vi "SR Test Launcher.vi"() -> ()   [LabVIEW 2018]
doc: "This VI is the launcher for the Car Wash Simulator.\n\nThis VI performs any actions required to occur before the modules begin running or after they close \n(such as creating the user events). \nIt then launches the modules. The UI is launched dynamically when the program is run."
uses:
  User Events/controls/Actions.ctl
  Modules/Error Handler/Error Handler.lvlib
  Modules/Base Controller/Controller.lvlib
  Modules/Database/Database.lvlib
panel:
  out "progress":u32(slide) scale=0.0..1500.0
  in  "error in":errorcluster
  out "error out":errorcluster
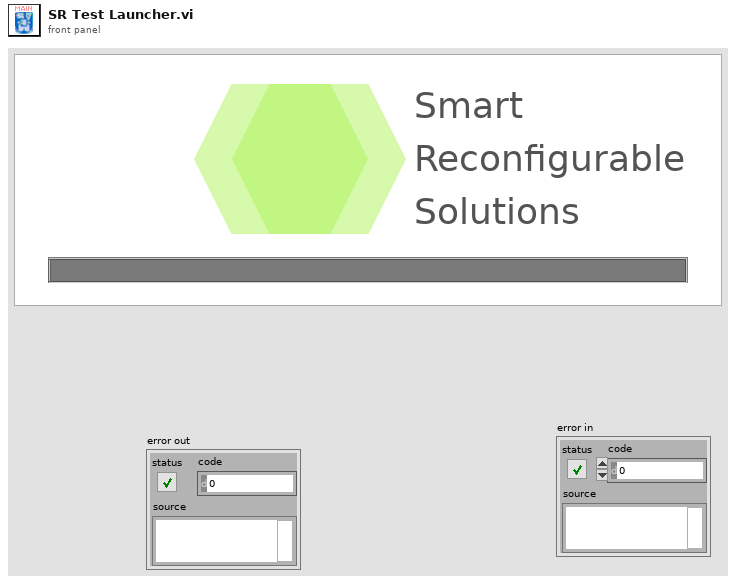
[diagram p1: front panel]
types:
  T1 = enum32{"Invalid", "Standard", "Closed", "Hidden", "Minimized", "Maximized"}
  T2 = typedef "Actions.ctl" = enum16{"Get", "Create", "Destroy"}
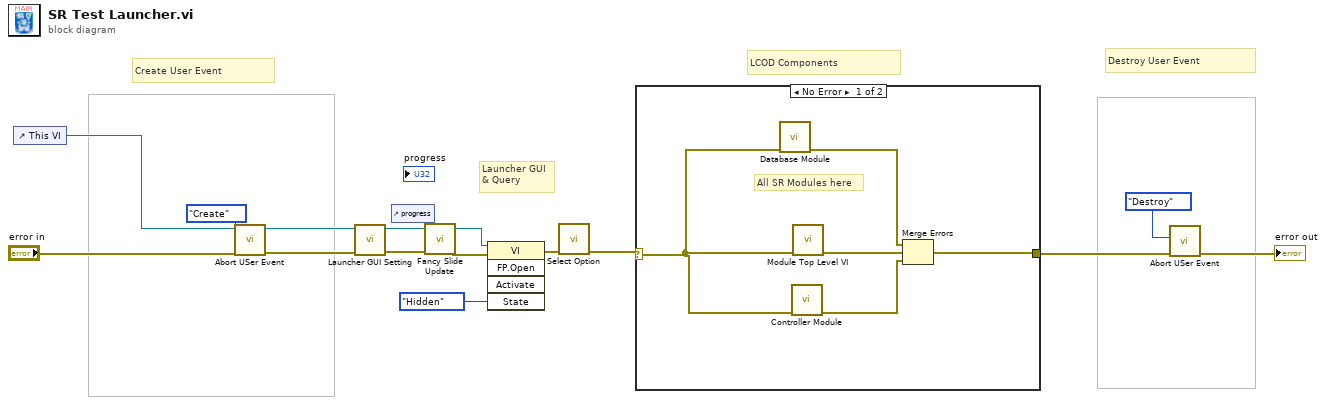
[diagram p0: block diagram]
diagram:
  # "Destroy User Event"
  # "LCOD Components"
  # "Create User Event"
  # "Launcher GUI\n& Query"
  n1 = control-ref of="This VI"() -> (w9:refnum<vi>)
  n2 = call "Abort USer Event.vi"("error in"="error in", "Enum"=Actions."Create") -> ("error out"=w10:errorcluster)  [unwired: 8 in, 1 out]
  n3 = call "Launcher GUI Setting.vi"("error in (no error)"=w10, "VI in"=w9) -> ("error out"=w6:errorcluster, "VI out"=w7:refnum<vi>)  [unwired: 8 in]
  n4 = control-ref of="progress"() -> (w4:refnum<vi>)
  n5 = call "Fancy Slide Update.vi"("error in (no error)"=w6, "Slide in"=w4) -> ("error out"=w1:errorcluster)  [unwired: 9 in]
  n6 = invoke class="VI" method="FP.Open"(reference=w7, error in=w1, "State"=T1."Hidden") -> (error out=w3:errorcluster)  [unwired: 2 in, 4 out]
  n7 = call "Select Option.vi"("error in"=w3) -> ("error out"=w2:errorcluster)  [unwired: 9 in, 1 out]
  n8 = case shown="No Error" w2 {
    selector: w2 -> [w16 w20]
    tunnel: [w18 w20] -> w13
    frame No Error {
      # "All SR Modules here"
      n9 = call "Database Module.vi"("error in"=w16) -> ("error out"=w15:errorcluster)  [unwired: 10 in]
      n10 = call "Controller Module.vi"("error in"=w16) -> ("error out"=w17:errorcluster)  [unwired: 10 in]
      n11 = call "Module Top Level VI.vi"("error in"=w16) -> ("error out"=w19:errorcluster)  [unwired: 10 in]
      n12 = Merge Errors(w15, w19, w17) -> (w18:errorcluster)
    }
    frame Error {
    }
  }
  n13 = call "Abort USer Event.vi"("error in"=w13, "Enum"=Actions."Destroy") -> ("error out"=→"error out":errorcluster)  [unwired: 8 in, 1 out]
